vi "二元一次方程.vi"(1 "B":dbl, 2 "X":dbl, 3 "K":dbl) -> (0 "Y":dbl)   [LabVIEW 2017]
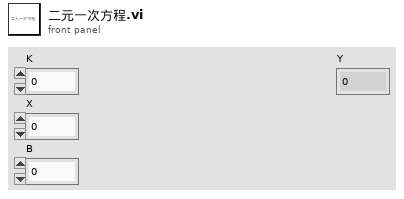
[diagram p1: front panel]
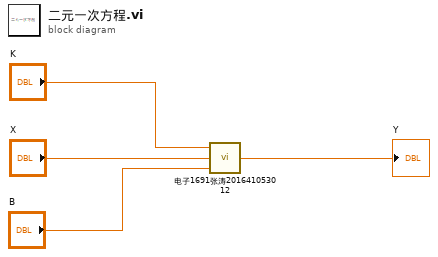
[diagram p0: block diagram]
diagram:
  n1 = call "电子1691张涛201641053012.vi"("B"="B", "X"="X", "K"="K") -> ("Y"=→"Y":dbl)
